vi "TestSimpleExpose.vi"   [LabVIEW 2017]
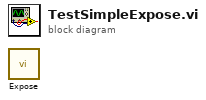
[diagram p0: block diagram]
diagram:
  n1 = call "Expose.vi"() -> ()  [unwired: 15 in, 1 out]
